vi "HFRR ADV v01.vi"() -> ()   [LabVIEW 2025] (continued)
                    n2104 = property on="Electrical Contact Resistance ( % )" class="WFChart (strict)"("History Data"=w3138) -> ()  [unwired: 2 in, 2 out]
                    n2105 = property on="Temperature ( Deg C )" class="WFChart (strict)"("History Data"=w3138) -> ()  [unwired: 2 in, 2 out]
                    n2106 = property on="Humidity ( %RH )" class="WFChart (strict)"("History Data"=w3138) -> ()  [unwired: 2 in, 2 out]
                    n2107 = property on="Stroke ( mm )" class="WFChart (strict)"("History Data"=w3139) -> ()  [unwired: 2 in, 2 out]
                    n2108 = property on="Stroke ( mm )" class="WFChart (strict)"("History Data"=w3139) -> ()  [unwired: 2 in, 2 out]
                    n2109 = local write "Humidity"(w3140) -> ()
                    n2110 = local write "Heater Button"(w3140) -> ()
                    n2111 = local read "FILE"() -> (w3134:string)
                    n2112 = disable-structure shown="Enabled" {
                      disable-tunnel: [w3179 _] -> w3125
                      frame Enabled {
                        n2113 = local read "NORMAL LOAD"() -> (w3179:dbl)
                      }
                      frame Disabled {
                      }
                    }
                    n2114 = call "file check.vi"("file name in"=w3134) -> ("error out"=w3137:errorcluster, "file name out"=w3131:string)  [unwired: 9 in]
                    n2115 = call "FILE PATH CREATION.vi"("error in"=w3137, "FILE NAME :"=w3131) -> ("FILE OUT"=w3130:path)  [unwired: 8 in, 1 out]
                    n2116 = Concatenate Strings(w3131, ".dgf" ("Substring")) -> (w3136:string)
                    n2117 = Concatenate Strings(w3131, ".duf" ("Substring")) -> (w3132:string)
                    n2118 = Multiply(x=w3125, y=1.0) -> (x*y=w3158:dbl)
                    n2119 = Build Path(base path=w3130, name or relative path=w3136) -> (appended path=w3129:path)
                    n2120 = Build Path(base path=w3130, name or relative path=w3132) -> (appended path=w3128:path)
                    n2121 = Number To Fractional String(number=w3158, width (-)=i16 5, precision (6)=i16 2) -> (F-format string=w3166:string)  [unwired: 1 in]
                    n2122 = local read "Fuel Discription :"() -> (w3154:string)
                    n2123 = local read "Batch Ref Num :"() -> (w3142:string)
                    n2124 = Get Date/Time String(date format (0)=enum16{"short", "long", "abbreviated"}."short") -> (date string=w3177:string, time string=w3174:string)  [unwired: 2 in]
                    n2125 = local read "Remarks :"() -> (w3153:string)
                    n2126 = Concatenate Strings("Load :- " ("Substring"), w3166, " grams ," ("Substring")) -> (w3165:string)
                    n2127 = local read "String 41"() -> (w3145:string)
                    n2128 = Concatenate Strings(w3154) -> (w3155:string)
                    n2129 = Concatenate Strings(w3142) -> (w3141:string)
                    n2130 = Concatenate Strings("tested by") -> (w3149:string)
                    n2131 = Concatenate Strings("(" ("Substring"), w3177, ")" ("Substring"), w3174) -> (w3147:string)
                    "concatenated string" <- w3147
                    n2132 = Concatenate Strings(w3153, "," ("string")) -> (w3152:string)
                    n2133 = Concatenate Strings("  TIME;      COF;       STROKE;     AIR TEMP;  TEMP;  HUMIDITY;  ECR; PID-OUT; FREQUENCY" ("Substring"), "\r") -> (w3161:string)
                    n2134 = Concatenate Strings(w3145, w3144, "Fuel Discription :-" ("Substring"), w3155, w3144, w3165, w3144, "Batch Ref Num :-" ("Substring"), w3141, w3144, " Remarks :- " ("Substring"), w3152, w3144, " Date :- " ("Substring"), w3147, w3144, "Tested By :-" ("Substring"), w3149) -> (w3159:string)
                    "REMARKS" <- w3159
                    n2135 = call <vilib>:"Write Characters To File.vi"("append to file? (new file:F)"=FALSE, "character string"=w3161, "file path (dialog if empty)"=w3129) -> ()  [unwired: 2 in, 1 out]
                    n2136 = call <vilib>:"Write Characters To File.vi"("append to file? (new file:F)"=FALSE, "character string"=w3159, "file path (dialog if empty)"=w3128) -> ()  [unwired: 2 in, 1 out]
                  }
                  frame #2 {
                    n2137 = local write "Cycles elapsed"(0 ("Cycles elapsed")) -> ()
                    n2138 = local write "cyclecount"(0 ("cyclecount")) -> ()
                    n2139 = local write "Save & Continue"(FALSE ("OK")) -> ()
                    n2140 = local write "autostrtflg"(TRUE ("autostrtflg")) -> ()
                    n2141 = local write "Save"(FALSE ("Save")) -> ()
                    n2142 = Get Date/Time In Seconds() -> (seconds since 1Jan1904=w3184:timestamp)
                    n2143 = To Double Precision Float(number=w3184) -> (double precision float=w3183:dbl)
                    n2144 = local write "acq timer"(w3183) -> ()
                    n2145 = One Button Dialog(message="Please ensure sample is mounted properly and machine is ready in all aspects for testing !", button name ("OK")="Ok") -> ()  [unwired: 1 out]
                  }
                  frame #3 {
                    n2146 = stacked-sequence {
                      frame #0 {
                        n2147 = local write "Main Dashboard Buttons"(T1."Dashboard" ("Main Dashboard Buttons")) -> ()
                        n2148 = local write "Main Tab"(T2."Acquire" ("Main Tab")) -> ()
                      }
                      frame #1 {
                        n2149 = local write "EVENT LOG"("" ("EVENT LOG")) -> ()
                      }
                      frame #2 {
                        n2150 = Wait (ms)(milliseconds to wait=u32 50) -> ()  [unwired: 1 out]
                      }
                      frame #3 {
                        n2151 = disable-structure shown="Disabled" {
                          frame Disabled {
                            n2152 = local read "EVENT LOG"() -> (w3196:string)
                            n2153 = call "Event Log.vi"("Content"="Test Details", "EVENT LOG"=w3196) -> ("EVENT LOG"=w3195:string)  [unwired: 8 in, 1 out]
                            n2154 = local write "EVENT LOG"(w3195) -> ()
                          }
                          frame Enabled {
                          }
                        }
                      }
                      frame #4 {
                        n2155 = Wait (ms)(milliseconds to wait=u32 50) -> ()  [unwired: 1 out]
                      }
                      frame #5 {
                        n2156 = local read "FILE"() -> (w3198:string)
                        n2157 = Concatenate Strings("File Name :" ("Content"), w3198) -> (w3199:string)
                        n2158 = local read "EVENT LOG"() -> (w3202:string)
                        n2159 = call "Event Log.vi"("Content"=w3199, "EVENT LOG"=w3202) -> ("EVENT LOG"=w3201:string)  [unwired: 8 in, 1 out]
                        n2160 = local write "EVENT LOG"(w3201) -> ()
                      }
                      frame #6 {
                        n2161 = Wait (ms)(milliseconds to wait=u32 50) -> ()  [unwired: 1 out]
                      }
                      frame #7 {
                        n2162 = local read "Batch Ref Num :"() -> (w3204:string)
                        n2163 = Concatenate Strings("Batch Ref No :" ("Content"), w3204) -> (w3205:string)
                        n2164 = local read "EVENT LOG"() -> (w3208:string)
                        n2165 = call "Event Log.vi"("Content"=w3205, "EVENT LOG"=w3208) -> ("EVENT LOG"=w3207:string)  [unwired: 8 in, 1 out]
                        n2166 = local write "EVENT LOG"(w3207) -> ()
                      }
                      frame #8 {
                        n2167 = Wait (ms)(milliseconds to wait=u32 50) -> ()  [unwired: 1 out]
                      }
                      frame #9 {
                        n2168 = local read "tested by"() -> (w3210:string)
                        n2169 = Concatenate Strings("Tested By :" ("Content"), w3210) -> (w3211:string)
                        n2170 = local read "EVENT LOG"() -> (w3214:string)
                        n2171 = call "Event Log.vi"("Content"=w3211, "EVENT LOG"=w3214) -> ("EVENT LOG"=w3213:string)  [unwired: 8 in, 1 out]
                        n2172 = local write "EVENT LOG"(w3213) -> ()
                      }
                      frame #10 {
                        n2173 = Wait (ms)(milliseconds to wait=u32 50) -> ()  [unwired: 1 out]
                      }
                      frame #11 {
                        n2174 = local read "TEST STANDARD"() -> (w3217:T3)
                        n2175 = case shown="\"ASTM D6079\", Default" w3217 {
                          tunnel: ["ASTM D6079" "ISO 12156" "CEC F-096-A-06" "Custom"] -> w3216
                          frame "ASTM D6079", Default {
                          }
                          frame "ISO 12156" {
                          }
                          frame "CEC F-096-A-06" {
                          }
                          frame "Custom" {
                          }
                        }
                        n2176 = Concatenate Strings("Test Standard :" ("Content"), w3216) -> (w3218:string)
                        n2177 = local read "EVENT LOG"() -> (w3221:string)
                        n2178 = call "Event Log.vi"("Content"=w3218, "EVENT LOG"=w3221) -> ("EVENT LOG"=w3220:string)  [unwired: 8 in, 1 out]
                        n2179 = local write "EVENT LOG"(w3220) -> ()
                      }
                      frame #12 {
                        n2180 = Wait (ms)(milliseconds to wait=u32 50) -> ()  [unwired: 1 out]
                      }
                      frame #13 {
                        n2181 = local read "Fuel Discription :"() -> (w3227:string)
                        n2182 = Concatenate Strings("Fuel Description :" ("Content"), w3227) -> (w3228:string)
                        n2183 = local read "EVENT LOG"() -> (w3231:string)
                        n2184 = call "Event Log.vi"("Content"=w3228, "EVENT LOG"=w3231) -> ("EVENT LOG"=w3230:string)  [unwired: 8 in, 1 out]
                        n2185 = local write "EVENT LOG"(w3230) -> ()
                      }
                      frame #14 {
                        n2186 = Wait (ms)(milliseconds to wait=u32 50) -> ()  [unwired: 1 out]
                      }
                      frame #15 {
                        n2187 = local read "Remarks :"() -> (w3233:string)
                        n2188 = Concatenate Strings("Remarks :" ("Content"), w3233) -> (w3234:string)
                        n2189 = local read "EVENT LOG"() -> (w3237:string)
                        n2190 = call "Event Log.vi"("Content"=w3234, "EVENT LOG"=w3237) -> ("EVENT LOG"=w3236:string)  [unwired: 8 in, 1 out]
                        n2191 = local write "EVENT LOG"(w3236) -> ()
                      }
                      frame #16 {
                        n2192 = Wait (ms)(milliseconds to wait=u32 50) -> ()  [unwired: 1 out]
                      }
                      frame #17 {
                        n2193 = local read "Operator ID"() -> (w3239:string)
                        n2194 = Concatenate Strings("Operator ID :" ("Content"), w3239) -> (w3241:string)
                        n2195 = local read "EVENT LOG"() -> (w3243:string)
                        n2196 = call "Event Log.vi"("Content"=w3241, "EVENT LOG"=w3243) -> ("EVENT LOG"=w3242:string)  [unwired: 8 in, 1 out]
                        n2197 = local write "EVENT LOG"(w3242) -> ()
                      }
                      frame #18 {
                        n2198 = Wait (ms)(milliseconds to wait=u32 50) -> ()  [unwired: 1 out]
                      }
                      frame #19 {
                        n2199 = disable-structure shown="Disabled" {
                          frame Disabled {
                            n2200 = local read "EVENT LOG"() -> (w3247:string)
                            n2201 = call "Event Log.vi"("Content"="Test Parameter", "EVENT LOG"=w3247) -> ("EVENT LOG"=w3246:string)  [unwired: 8 in, 1 out]
                            n2202 = local write "EVENT LOG"(w3246) -> ()
                          }
                          frame Enabled {
                          }
                        }
                      }
                      frame #20 {
                        n2203 = Wait (ms)(milliseconds to wait=u32 50) -> ()  [unwired: 1 out]
                      }
                      frame #21 {
                        n2204 = local read "Set Hz"() -> (w3251:dbl)
                        n2205 = Number To Fractional String(number=w3251, precision (6)=i16 2) -> (F-format string=w3250:string)  [unwired: 2 in]
                        n2206 = Concatenate Strings("Set Frequency [Hz] :" ("Content"), w3250) -> (w3253:string)
                        n2207 = local read "EVENT LOG"() -> (w3255:string)
                        n2208 = call "Event Log.vi"("Content"=w3253, "EVENT LOG"=w3255) -> ("EVENT LOG"=w3254:string)  [unwired: 8 in, 1 out]
                        n2209 = local write "EVENT LOG"(w3254) -> ()
                      }
                      frame #22 {
                        n2210 = Wait (ms)(milliseconds to wait=u32 50) -> ()  [unwired: 1 out]
                      }
                      frame #23 {
                        n2211 = local read "NORMAL LOAD"() -> (w3258:dbl)
                        n2212 = Number To Fractional String(number=w3258, precision (6)=i16 2) -> (F-format string=w3259:string)  [unwired: 2 in]
                        n2213 = Concatenate Strings("Applied Load [grams] :" ("Content"), w3259) -> (w3261:string)
                        n2214 = local read "EVENT LOG"() -> (w3263:string)
                        n2215 = call "Event Log.vi"("Content"=w3261, "EVENT LOG"=w3263) -> ("EVENT LOG"=w3262:string)  [unwired: 8 in, 1 out]
                        n2216 = local write "EVENT LOG"(w3262) -> ()
                      }
                      frame #24 {
                        n2217 = Wait (ms)(milliseconds to wait=u32 50) -> ()  [unwired: 1 out]
                      }
                      frame #25 {
                        n2218 = local read "Set Strk"() -> (w3266:dbl)
                        n2219 = Number To Fractional String(number=w3266, precision (6)=i16 2) -> (F-format string=w3267:string)  [unwired: 2 in]
                        n2220 = Concatenate Strings("Set Stroke [mm] :" ("Content"), w3267) -> (w3269:string)
                        n2221 = local read "EVENT LOG"() -> (w3271:string)
                        n2222 = call "Event Log.vi"("Content"=w3269, "EVENT LOG"=w3271) -> ("EVENT LOG"=w3270:string)  [unwired: 8 in, 1 out]
                        n2223 = local write "EVENT LOG"(w3270) -> ()
                      }
                      frame #26 {
                        n2224 = Wait (ms)(milliseconds to wait=u32 50) -> ()  [unwired: 1 out]
                      }
                      frame #27 {
                        n2225 = local read "Set Temp"() -> (w3274:dbl)
                        n2226 = Number To Fractional String(number=w3274, precision (6)=i16 2) -> (F-format string=w3275:string)  [unwired: 2 in]
                        n2227 = Concatenate Strings("Set Temperature [deg C] :" ("Content"), w3275) -> (w3277:string)
                        n2228 = local read "EVENT LOG"() -> (w3279:string)
                        n2229 = call "Event Log.vi"("Content"=w3277, "EVENT LOG"=w3279) -> ("EVENT LOG"=w3278:string)  [unwired: 8 in, 1 out]
                        n2230 = local write "EVENT LOG"(w3278) -> ()
                      }
                      frame #28 {
                        n2231 = Wait (ms)(milliseconds to wait=u32 50) -> ()  [unwired: 1 out]
                      }
                      frame #29 {
                        n2232 = local read "Set Rh"() -> (w3282:dbl)
                        n2233 = Number To Fractional String(number=w3282, precision (6)=i16 2) -> (F-format string=w3283:string)  [unwired: 2 in]
                        n2234 = Concatenate Strings("Set Humidity [%RH] :" ("Content"), w3283) -> (w3285:string)
                        n2235 = local read "EVENT LOG"() -> (w3287:string)
                        n2236 = call "Event Log.vi"("Content"=w3285, "EVENT LOG"=w3287) -> ("EVENT LOG"=w3286:string)  [unwired: 8 in, 1 out]
                        n2237 = local write "EVENT LOG"(w3286) -> ()
                      }
                      frame #30 {
                        n2238 = Wait (ms)(milliseconds to wait=u32 50) -> ()  [unwired: 1 out]
                      }
                      frame #31 {
                        n2239 = local read "test time"() -> (w3290:dbl)
                        n2240 = Number To Fractional String(number=w3290, precision (6)=i16 1) -> (F-format string=w3291:string)  [unwired: 2 in]
                        n2241 = Concatenate Strings("Test Duration [mins] :" ("Content"), w3291) -> (w3293:string)
                        n2242 = local read "EVENT LOG"() -> (w3295:string)
                        n2243 = call "Event Log.vi"("Content"=w3293, "EVENT LOG"=w3295) -> ("EVENT LOG"=w3294:string)  [unwired: 8 in, 1 out]
                        n2244 = local write "EVENT LOG"(w3294) -> ()
                      }
                      frame #32 {
                        w3296 = dbl[] [] ("History Data")
                        w3297 = cluster{"y":dbl, dbl, "y":dbl}[] [] ("History Data")
                        w3298 = FALSE ("Visible")
                        n2245 = property on="Stroke ( mm )" class="WFChart (strict)"("History Data"=w3297) -> ()  [unwired: 2 in, 2 out]
                        n2246 = property on="Humidity ( %RH )" class="WFChart (strict)"("History Data"=w3296) -> ()  [unwired: 2 in, 2 out]
                        n2247 = property on="Temperature ( Deg C )" class="WFChart (strict)"("History Data"=w3296) -> ()  [unwired: 2 in, 2 out]
                        n2248 = property on="Electrical Contact Resistance ( % )" class="WFChart (strict)"("History Data"=w3296) -> ()  [unwired: 2 in, 2 out]
                        n2249 = property on="Coefficient of Friction" class="WFChart (strict)"("History Data"=w3296) -> ()  [unwired: 2 in, 2 out]
                        n2250 = property on="Frictional Force ( N )" class="WFChart (strict)"("History Data"=w3296) -> ()  [unwired: 2 in, 2 out]
                        n2251 = property on="Coefficient of Friction" class="WFChart (strict)"("History Data"=w3296) -> ()  [unwired: 2 in, 2 out]
                        n2252 = property on="Frictional Force ( N )" class="WFChart (strict)"("History Data"=w3296) -> ()  [unwired: 2 in, 2 out]
                        n2253 = property on="Electrical Contact Resistance ( % )" class="WFChart (strict)"("History Data"=w3296) -> ()  [unwired: 2 in, 2 out]
                        n2254 = property on="Humidity ( %RH )" class="WFChart (strict)"("History Data"=w3296) -> ()  [unwired: 2 in, 2 out]
                        n2255 = property on="Stroke ( mm )" class="WFChart (strict)"("History Data"=w3297) -> ()  [unwired: 2 in, 2 out]
                        n2256 = property on="Temperature ( Deg C )" class="WFChart (strict)"("History Data"=w3296) -> ()  [unwired: 2 in, 2 out]
                        n2257 = property on="Service Password Log" class="Str"("Visible"=w3298) -> ()  [unwired: 2 in, 2 out]
                        n2258 = property on="Password 3" class="Clust (strict)"("Visible"=w3298) -> ()  [unwired: 2 in, 2 out]
                      }
                    }
                    "TEST FILE NAM,E SAVED" <- TRUE ("TEST FILE NAM,E SAVED")
                  }
                }
              }
            }
          }
        }
        n2259 = case shown="True" w2614 {
          frame False {
            n2260 = local write "tfalg"(0.0 ("tfalg")) -> ()
          }
          frame True {
            n2261 = local read "tfalg"() -> (w2759:dbl)
            n2262 = Equal?(x=w2759, y=0.0) -> (x = y?=w2760:bool)
            n2263 = case shown="True" w2760 {
              frame False {
              }
              frame True {
                n2264 = local read "Total No. of Tests"() -> (w2763:dbl)
                n2265 = local write "tfalg"(1.0 ("tfalg")) -> ()
                n2266 = local write "acq 2"(FALSE ("acq 2")) -> ()
                n2267 = Wait (ms)(milliseconds to wait=u32 200) -> ()  [unwired: 1 out]
                n2268 = Increment(x=w2763) -> (x+1=w2762:dbl)
                n2269 = local write "Total No. of Tests"(w2762) -> ()
              }
            }
          }
        }
        n2270 = local write "Test \nStatus"(w2620) -> ()
        n2271 = local write "Save"(w2620) -> ()
        n2272 = local read "Main Tab"() -> (w2577:T2)
        n2273 = case shown="True" w2601 {
          tunnel: [FALSE ("RUN") TRUE ("RUN")] -> w2600
          tunnel: [_ 1] -> w2593
          frame False {
          }
          frame True {
          }
        }
        n2274 = In Range and Coerce(upper limit=w2608, x=w2581, lower limit=w2607) -> (In Range?=w2599:bool)  [unwired: 1 out]
        n2275 = In Range and Coerce(upper limit=w2605, x=w2580, lower limit=w2606) -> (In Range?=w2597:bool)  [unwired: 1 out]
        n2276 = case shown="True" w2613 {
          frame False {
            n2277 = local read "Rt 3"() -> (w2741:bool)
            n2278 = case shown="True" w2741 {
              frame False {
              }
              frame True {
                n2279 = local write "Rt 3"(FALSE ("Rt 3")) -> ()
                n2280 = local write "Json End Flg"(TRUE ("Upld AR 2")) -> ()
              }
            }
            "Rt" <- TRUE ("Rt")
            "Rt 2" <- FALSE ("Rt")
          }
          frame True {
            n2281 = local read "Rt"() -> (w2748:bool)
            n2282 = local write "Rt 2"(TRUE ("Rt 2")) -> ()
            n2283 = case shown="True" w2748 {
              frame False {
              }
              frame True {
                w2749 = TRUE ("Upld AR 2")
                n2284 = local write "Rt"(FALSE ("Rt")) -> ()
                n2285 = local write "Upld AR"(w2749) -> ()
                n2286 = local write "Json St Flg"(w2749) -> ()
              }
            }
            "Rt 3" <- TRUE ("Rt 3")
          }
        }
        n2287 = case shown="True" w2599 {
          tunnel: [FALSE ("RUN") TRUE ("RUN")] -> w2598
          tunnel: [_ 2] -> w2592
          frame False {
          }
          frame True {
          }
        }
        n2288 = case shown="True" w2597 {
          tunnel: [FALSE ("RUN") TRUE ("RUN")] -> w2596
          tunnel: [_ 3] -> w2591
          frame False {
          }
          frame True {
          }
        }
        n2289 = case shown="\"Acquire\"" w2577 {
          tunnel: w2579 -> [_ w2810]
          frame Default {
            w2809 = 0.0 ("output")
            n2290 = local write "PID-out"(w2809) -> ()
            n2291 = local write "Frequency ( Hz )"(w2809) -> ()
          }
          frame "Acquire" {
            n2292 = stacked-sequence {
              frame #0 {
                n2293 = local read "Auto Start Test"() -> (w2812:bool)
                n2294 = case shown="True" w2812 {
                  tunnel: "RUN" -> [w2833 w2836]
                  tunnel: [w2833 w2835] -> w2813
                  frame False {
                  }
                  frame True {
                    n2295 = local read "Auto Start Temp"() -> (w2834:bool)
                    n2296 = Or(x=w2836, y=w2834) -> (x .or. y?=w2835:bool)
                  }
                }
                n2297 = local read "clk"() -> (w2832:dbl)
                n2298 = local read "Save"() -> (w2828:bool)
                n2299 = Equal?(x=w2832, y=0.0) -> (x = y?=w2829:bool)
                n2300 = And(x=w2829, y=w2828) -> (x .and. y?=w2830:bool)
                n2301 = Not(x="Engage") -> (.not. x?=w2819:bool)
                n2302 = case shown="False" w2813 {
                  tunnel: [0.0 w2860] -> w2815
                  frame False {
                    (unwired) TRUE ("Visible")
                    n2303 = local read "Auto Start Test"() -> (w2840:bool)
                    n2304 = local write "Start Time"(TRUE ("Start Time")) -> ()
                    n2305 = property on="Stroke 2" class="DigNum (strict)"("Visible"=FALSE) -> ()  [unwired: 2 in, 2 out]
                    n2306 = case shown="False" w2840 {
                      frame False {
                        n2307 = property on="Heater Button" class="Bool (strict)"("DisabledEnum"=T15."Enabled" ("Disabled")) -> ()  [unwired: 2 in, 2 out]
                        n2308 = property on="Humidity" class="Bool (strict)"("DisabledEnum"=T15."Enabled" ("Disabled")) -> ()  [unwired: 2 in, 2 out]
                      }
                      frame True {
                      }
                    }
                    n2309 = case shown="False" "TestCompFlg" {
                      frame False {
                        n2310 = local read "StartFlg"() -> (w2848:bool)
                        n2311 = case shown="True" w2848 {
                          frame False {
                          }
                          frame True {
                            n2312 = flat-sequence {
                              frame #0 {
                                n2313 = local read "EVENT LOG"() -> (w2850:string)
                                n2314 = call "Event Log.vi"("Content"="Test was interrupted", "EVENT LOG"=w2850) -> ("EVENT LOG"=w2851:string)  [unwired: 8 in, 1 out]
                                n2315 = local write "EVENT LOG"(w2851) -> ()
                              }
                              frame #1 {
                                w2852 = FALSE ("StartFlg")
                                n2316 = local write "Heater Button"(w2852) -> ()
                                n2317 = local write "StartFlg"(w2852) -> ()
                                n2318 = local write "Humidity"(w2852) -> ()
                              }
                            }
                          }
                        }
                      }
                      frame True {
                      }
                    }
                    n2319 = local write "String 14"("Test will autostart once parameters reach the set value." ("String 14")) -> ()
                  }
                  frame True {
                    (unwired) FALSE ("Visible")
                    n2320 = property on="Stroke 2" class="DigNum (strict)"("Visible"=TRUE) -> ()  [unwired: 2 in, 2 out]
                    n2321 = property on="STOP 2" class="Bool (strict)"("Disabled"=u8 2) -> ()  [unwired: 2 in, 2 out]
                    n2322 = local write "String 14"(" Running....." ("String 14")) -> ()
                    n2323 = property on="Heater Button" class="Bool (strict)"("DisabledEnum"=T15."Disabled and Grayed Out" ("Disabled")) -> ()  [unwired: 2 in, 2 out]
                    n2324 = property on="Humidity" class="Bool (strict)"("DisabledEnum"=T15."Disabled and Grayed Out" ("Disabled")) -> ()  [unwired: 2 in, 2 out]
                    n2325 = case shown="True" "Start Time" {
                      selector: "Start Time" -> [_ w2870]
                      frame False {
                      }
                      frame True {
                        n2326 = Not(x=w2870) -> (.not. x?=w2869:bool)
                        n2327 = local write "Start Time"(w2869) -> ()
                        n2328 = local read "EVENT LOG"() -> (w2871:string)
                        n2329 = call "Event Log.vi"("Content"="Test in progress", "EVENT LOG"=w2871) -> ("EVENT LOG"=w2873:string)  [unwired: 8 in, 1 out]
                        n2330 = local write "EVENT LOG"(w2873) -> ()
                      }
                    }
                    n2331 = local read "Set Hz"() -> (w2867:dbl)
                    n2332 = call <vilib>:"Uniform White Noise Waveform.vi"() -> ("signal out"=w2866:waveform(dbl))  [unwired: 10 in, 1 out]
                    n2333 = local read "Freq"() -> (w2859:dbl)
                    n2334 = Add(x=w2867, y=w2866) -> (x+y=w2865:waveform(dbl))
                    n2335 = Multiply(x=w2865, y=ext 0.1) -> (x*y=w2861:waveform(ext))
                    n2336 = Multiply(x=w2859, y=0.9) -> (x*y=w2862:dbl)
                    n2337 = Add(x=w2861, y=w2862) -> (x+y=w2860:waveform(ext))
                    "StartFlg" <- TRUE ("StartFlg")
                  }
                }
                n2338 = case shown="True" w2830 {
                  frame False {
                  }
                  frame True {
                    n2339 = local write "clk"(10.0 ("clk")) -> ()
                    n2340 = Get Date/Time In Seconds() -> (seconds since 1Jan1904=w2876:timestamp)
                    n2341 = To Double Precision Float(number=w2876) -> (double precision float=w2874:dbl)
                    n2342 = local write "acq timer"(w2874) -> ()
                    n2343 = local write "act save time"(w2874) -> ()
                  }
                }
                n2344 = call "Elapsed Time"("Time Target (s)"="Countdown", "Reset"=w2819) -> ("Elapsed Time (s)"=w2824:dbl, "Time has Elapsed"=w2822:bool)  [unwired: 10 in, 6 out]
                "Countdown 2" <- w2824
                n2345 = Subtract(x=w2824, y=2.0) -> (x-y=w2827:dbl)
                n2346 = Less?(x=w2827, y="Countdown") -> (x < y?=w2825:bool)
                n2347 = And(x=w2825, y=w2822) -> (x .and. y?=w2821:bool)
                n2348 = case shown="True" w2821 {
                  frame False {
                  }
                  frame True {
                    (unwired) dbl[] [] ("History Data")
                    n2349 = local write "Engage"(FALSE ("Engage")) -> ()
                    n2350 = local write "RUN"(TRUE ("RUN")) -> ()
                    n2351 = local read "Humidity ( %RH )"() -> (→"Rh Before":dbl)
                  }
                }
                n2352 = local read "Test \nStatus"() -> (w2817:bool)
                n2353 = Select(t=w2815, s=w2817, f=0.0) -> (s? t:f=w2816:dbl)
                n2354 = local write "Frequency ( Hz )"(w2816) -> ()
                n2355 = local write "Freq"(w2816) -> ()
              }
              frame #1 {
                w2899 = 1000000.0 ("x")
                # "Elapsed time\ncof\nstroke\nAir temp\nTemp\nHumidity"
                # "acq timer\n\nact save time"
                # "convert to microseconds"
                n2356 = local read "COUNT"() -> (w2882:i32)
                n2357 = local read "Rate"() -> (w2895:dbl)
                n2358 = Divide(x=w2899, y=w2895) -> (x/y=w2900:dbl)
                n2359 = Greater Or Equal?(x=w2882, y=250) -> (x >= y?=w2881:bool)
                n2360 = Get Date/Time In Seconds() -> (seconds since 1Jan1904=w2902:timestamp)
                n2361 = case shown="True" w2881 {
                  frame False {
                    n2362 = local read "COUNT"() -> (w2903:i32)
                    n2363 = Increment(x=w2903) -> (x+1=w2904:i32)
                    n2364 = local write "COUNT"(w2904) -> ()
                  }
                  frame True {
                    n2365 = local write "COUNT"(0 ("COUNT")) -> ()
                  }
                }
                n2366 = local read "Samplingtime 2"() -> (w2880:dbl)
                n2367 = local read "act save time"() -> (w2897:dbl)
                n2368 = Divide(x=w2900, y=w2899) -> (x/y=w2898:dbl)
                n2369 = To Double Precision Float(number=w2902) -> (double precision float=w2891:dbl)
                n2370 = Add(x=w2897, y=w2880) -> (x+y=w2896:dbl)
                n2371 = local read "acq timer"() -> (w2901:dbl)
                n2372 = local read "COUNT"() -> (w2884:i32)
                n2373 = Greater Or Equal?(x=w2891, y=w2896) -> (x >= y?=w2879:bool)
                n2374 = Multiply(x=w2898, y=w2884) -> (x*y=w2890:dbl)
                n2375 = Subtract(x=w2891, y=w2901) -> (x-y=w2893:dbl)
                n2376 = local read "Save"() -> (w2894:bool)
                n2377 = Add(x=w2893, y=w2890) -> (x+y=w2877:dbl)
                "Elapsed time 3" <- w2877
                n2378 = And(x=w2879, y=w2894) -> (x .and. y?=w2892:bool)
                n2379 = Divide(x=w2877, y=60.0) -> (x/y=w2888:dbl)
                n2380 = local read "Test \nStatus"() -> (w2878:bool)
                n2381 = local read "clk"() -> (w2885:dbl)
                n2382 = Equal?(x=w2885, y=10.0) -> (x = y?=w2887:bool)
                n2383 = case shown="True" w2892 {
                  tunnel: w2891 -> [_ w3001]
                  tunnel: [FALSE ("Boolean 2") TRUE ("Boolean 2")] -> _
                  frame False {
                  }
                  frame True {
                    w2955 = ";" ("Substring")
                    # "Pid out/\nFreq response value"
                    n2384 = local write "act save time"(w3001) -> ()
                    n2385 = local read "FILE"() -> (w2949:string)
                    n2386 = call "file check.vi"("file name in"=w2949) -> ("error out"=w2952:errorcluster, "file name out"=w2947:string)  [unwired: 9 in]
                    n2387 = call "FILE PATH CREATION.vi"("error in"=w2952, "FILE NAME :"=w2947) -> ("FILE OUT"=w2950:path)  [unwired: 8 in, 1 out]
                    n2388 = Concatenate Strings(w2947, ".dgf" ("Substring")) -> (w2951:string)
                    n2389 = local read "FF 2"() -> (→"Frictional Force ( N )" →"Frictional Force ( N )":dbl)
                    n2390 = Build Path(base path=w2950, name or relative path=w2951) -> (appended path=w2946:path)
                    n2391 = local read "COF 2"() -> (w2960:dbl)
                    "cof" <- w2960
                    "Coefficient of Friction" <- w2960
                    "COF 4" <- w2960
                    "Coefficient of Friction" <- w2960
                    n2392 = local read "TEMP"() -> (w2963:dbl)
                    "Temp" <- w2963
                    "Temperature ( Deg C )" <- w2963
                    n2393 = local read "Humidity ( %RH )"() -> (w2962:dbl)
                    "Humidity ( %RH )" <- w2962
                    "Humidity ( %RH )" <- w2962
                    n2394 = local read "Frequency ( Hz )"() -> (w2969:dbl)
                    n2395 = local read "Elapsed time"() -> (w2994:dbl)
                    n2396 = local read "AIR TEMP"() -> (w2967:dbl)
                    n2397 = local read "PID-out"() -> (w2972:dbl)
                    n2398 = local write "Temperature ( Deg C )"(w2963) -> ()
                    n2399 = Number To Fractional String(number="measured_stroke", width (-)=i16 9 ("precision (6)"), precision (6)=i16 6) -> (F-format string=w2987:string)  [unwired: 1 in]
                    n2400 = Number To Fractional String(number=w2967, width (-)=i16 9 ("precision (6)"), precision (6)=i16 3) -> (F-format string=w2986:string)  [unwired: 1 in]
                    n2401 = Number To Fractional String(number=w2963, width (-)=i16 9 ("precision (6)"), precision (6)=i16 3) -> (F-format string=w2983:string)  [unwired: 1 in]
                    n2402 = Number To Fractional String(number=w2962, width (-)=i16 9 ("precision (6)"), precision (6)=i16 3) -> (F-format string=w2980:string)  [unwired: 1 in]
                    n2403 = Number To Fractional String(number=0.0, width (-)=i16 9 ("precision (6)"), precision (6)=i16 3) -> (F-format string=w2977:string)  [unwired: 1 in]
                    n2404 = Number To Fractional String(number=w2972, width (-)=i16 9 ("precision (6)"), precision (6)=i16 3) -> (F-format string=w2973:string)  [unwired: 1 in]
                    n2405 = Number To Fractional String(number=w2969, width (-)=i16 9 ("precision (6)"), precision (6)=i16 3) -> (F-format string=w2968:string)  [unwired: 1 in]
                    n2406 = Number To Fractional String(number=w2960, width (-)=i16 9 ("precision (6)"), precision (6)=i16 6) -> (F-format string=w2995:string)  [unwired: 1 in]
                    n2407 = Number To Fractional String(number=w2994, width (-)=i16 14 ("precision (6)"), precision (6)=i16 3) -> (F-format string=w2996:string)  [unwired: 1 in]
                    n2408 = Bundle("y"=1.02, "measured_stroke"="measured_stroke", "y"=0.98) -> (w2961:cluster{"y":dbl, "measured_stroke":dbl, "y":dbl})  [unwired: 1 in]
                    n2409 = Number To Fractional String(number="Ambient Humidity :", width (-)=i16 9 ("precision (6)"), precision (6)=i16 6) -> (F-format string=w2953:string)  [unwired: 1 in]
                    n2410 = local read "RUN"() -> (w2959:bool)
                    n2411 = case shown="True" w2959 {
                      tunnel: w2961 -> [_ w3006]
                      tunnel: "measured_stroke" -> [_ w3005]
                      tunnel: "measured_stroke" -> [_ w3004]
                      tunnel: "measured_stroke" -> [_ w3003]
                      frame False {
                      }
                      frame True {
                        "Stroke ( mm )" <- w3006
                        "Stroke ( mm )" <- w3006
                        "Stroke 4" <- w3005
                        "Stroke 3" <- w3004
                        "Stroke 2" <- w3003
                      }
                    }
                    n2412 = Concatenate Strings(w2996, w2955, w2995, w2955, w2987, w2955, w2986, w2955, w2983, w2955, w2980, w2955, w2977, w2955, w2973, w2955, w2968, w2955, w2953, "\r") -> (w2993:string)
                    n2413 = call <vilib>:"Write Characters To File.vi"("append to file? (new file:F)"=TRUE, "character string"=w2993, "file path (dialog if empty)"=w2946) -> ()  [unwired: 2 in, 1 out]
                    "refresh flag" <- TRUE ("refresh flag")
                  }
                }
                n2414 = case shown="True" w2878 {
                  tunnel: w2888 -> [_ w2914]
                  tunnel: w2893 -> [_ w2924]
                  tunnel: [0.0 w2920] -> _
                  tunnel: w2887 -> [_ w2919]
                  tunnel: [0.0 w2918] -> _
                  tunnel: w2877 -> [_ w2918]
                  tunnel: w2891 -> [w2907 _]
                  frame False {
                    n2415 = local write "acq timer"(w2907) -> ()
                    n2416 = local write "Test Duration Status"(0.0 ("Test Duration Status")) -> ()
                  }
                  frame True {
                    n2417 = local read "Set Hz"() -> (w2921:dbl)
                    n2418 = local write "Elapsed time"(w2914) -> ()
                    n2419 = local read "test time"() -> (w2913:dbl)
                    n2420 = Multiply(x=w2924, y=w2921) -> (x*y=w2923:dbl)
                    n2421 = case shown="False" w2919 {
                      tunnel: w2923 -> [w2925 _]
                      tunnel: [w2925 1.0] -> w2920
                      frame False {
                        n2422 = local write "Cycles elapsed"(w2925) -> ()
                      }
                      frame True {
                      }
                    }
                    n2423 = Greater?(x=w2914, y=w2913) -> (0:w2922:bool)
                    n2424 = Subtract(x=w2913, y=w2914) -> (x-y=w2912:dbl)
                    "time" <- w2912
                    n2425 = Multiply(x=w2912, y=60.0) -> (x*y=w2911:dbl)
                    n2426 = local write "Time Remaining"(w2911) -> ()
                    n2427 = local write "Remaining Time"(w2911) -> ()
                    n2428 = case shown="True" w2922 {
                      frame False {
                      }
                      frame True {
                        w2927 = T15."Enabled" ("Disabled")
                        w2931 = "" ("FILE")
                        w2932 = TRUE ("Visible")
                        n2429 = local write "Humidity"(FALSE ("Humidity")) -> ()
                        n2430 = local write "RUN"(FALSE ("OK Button 2")) -> ()
                        n2431 = local write "Heater Button"(FALSE ("Heater Button")) -> ()
                        n2432 = local write "Auto Start Test"(FALSE ("Auto Start Test")) -> ()
                        n2433 = local write "TestCompFlg"(TRUE ("StpFlg")) -> ()
                        n2434 = local read "Humidity ( %RH )"() -> (→"Rh After":dbl)
                        n2435 = property on="STOP 2" class="Bool (strict)"("Disabled"=u8 0) -> ()  [unwired: 2 in, 2 out]
                        n2436 = local read "EVENT LOG"() -> (w2937:string)
                        n2437 = call "Event Log.vi"("Content"="Test Completed", "EVENT LOG"=w2937) -> ("EVENT LOG"=w2936:string)  [unwired: 8 in, 1 out]
                        n2438 = property on="RUN" class="Bool (strict)"("Visible"=w2932) -> ()  [unwired: 2 in, 2 out]
                        n2439 = property on="Auto Start Test" class="Bool (strict)"("Visible"=w2932) -> ()  [unwired: 2 in, 2 out]
                        n2440 = local write "Batch Ref Num :"(w2931) -> ()
                        n2441 = local write "FILE"(w2931) -> ()
                        n2442 = local write "EVENT LOG"(w2936) -> ()
                        n2443 = local write "TEST FILE NAM,E SAVED"(FALSE ("TEST FILE NAM,E SAVED")) -> ()
                        n2444 = local write "Fuel Discription :"(w2931) -> ()
                        n2445 = local write "Remarks :"(w2931) -> ()
                        n2446 = local write "Main Dashboard Buttons"(T1."Imaging" ("Main Dashboard Buttons")) -> ()
                        n2447 = local write "Main Tab"(T2."Adv Scar" ("Main Tab")) -> ()
                        n2448 = property on="FRICVALZ 2" class="Bool (strict)"("DisabledEnum"=w2927) -> ()  [unwired: 2 in, 2 out]
                        n2449 = property on="FRICVALZ 3" class="Bool (strict)"("DisabledEnum"=w2927) -> ()  [unwired: 2 in, 2 out]
                        n2450 = property on="FRICVALZ 4" class="Bool (strict)"("DisabledEnum"=w2927) -> ()  [unwired: 2 in, 2 out]
                      }
                    }
                    n2451 = Divide(x=w2914, y=w2913) -> (x/y=w2917:dbl)
                    n2452 = Multiply(x=w2917, y=100.0) -> (x*y=w2915:dbl)
                    n2453 = local write "Test Duration Status"(w2915) -> ()
                  }
                }
              }
              frame #2 {
                n2454 = case shown="True" "Heater Button" {
                  tunnel: [0.0 ("output") w3030] -> w3007
                  frame False {
                    w3010 = TRUE ("tmpchk")
                    n2455 = local read "TEMP"() -> (w3011:dbl)
                    n2456 = local write "Temp ini"(w3011) -> ()
                    n2457 = local write "Reset 4"(w3010) -> ()
                    n2458 = local write "tmpchk"(w3010) -> ()
                    n2459 = local write "reinit"(TRUE ("reinit")) -> ()
                    n2460 = local write "manual temp log"(TRUE ("manual temp log")) -> ()
                  }
                  frame True {
                    # "Logic to turn off\nthe heater when \ntemp is not rising.\nTime - 60 sec\nDelta t- 5°c"
                    n2461 = local read "Temp ini"() -> (w3018:dbl)
                    n2462 = local read "Auto Start Test"() -> (w3014:bool)
                    n2463 = Less?(x=w3018, y=53.0) -> (x < y?=w3016:bool)
                    n2464 = case shown="False" w3014 {
                      frame False {
                        n2465 = local read "Set Temp"() -> (w3041:dbl)
                        n2466 = local read "TEMP"() -> (w3040:dbl)
                        n2467 = Subtract(x=w3041, y=w3040) -> (x-y=w3039:dbl)
                        n2468 = Absolute Value(x=w3039) -> (abs(x)=w3038:dbl)
                        n2469 = Less?(x=w3038, y=0.5) -> (x < y?=w3036:bool)
                        n2470 = case shown="True" w3036 {
                          tunnel: "manual temp log" -> [_ w3042]
                          frame False {
                          }
                          frame True {
                            n2471 = case shown="True" w3042 {
                              selector: w3042 -> [_ w3043]
                              frame False {
                              }
                              frame True {
                                # "#Event log"
                                n2472 = Not(x=w3043) -> (.not. x?=w3044:bool)
                                n2473 = local write "manual temp log"(w3044) -> ()
                                n2474 = local read "EVENT LOG"() -> (w3047:string)
                                n2475 = call "Event Log.vi"("Content"="Target Temperature reached", "EVENT LOG"=w3047) -> ("EVENT LOG"=w3046:string)  [unwired: 8 in, 1 out]
                                n2476 = local write "EVENT LOG"(w3046) -> ()
                              }
                            }
                          }
                        }
                      }
                      frame True {
                        n2477 = local write "manual temp log"(TRUE ("manual temp log")) -> ()
                      }
                    }
                    n2478 = And(x="tmpchk", y=w3016) -> (x .and. y?=w3019:bool)
                    n2479 = case shown="True" w3019 {
                      frame False {
                      }
                      frame True {
                        n2480 = call "Elapsed Time8"("Time Target (s)"=300.0, "Reset"="Reset 4") -> ("Time has Elapsed"=w3049:bool)  [unwired: 10 in, 7 out]
                        n2481 = flat-sequence {
                          tunnel: w3049 -> [_]
                          frame #0 {
                            n2482 = local write "Reset 4"(FALSE ("Reset 4")) -> ()
                          }
                        }
                        n2483 = case shown="True" w3049 {
                          frame False {
                          }
                          frame True {
                            n2484 = local read "Temp ini"() -> (w3056:dbl)
                            n2485 = Add(x=w3056, y=5.0) -> (x+y=w3054:dbl)
                            n2486 = local read "TEMP"() -> (w3057:dbl)
                            n2487 = Greater?(x=w3057, y=w3054) -> (0:w3055:bool)
                            n2488 = case shown="False" w3055 {
                              frame False {
                                n2489 = local write "Heater Button"(FALSE ("Heater Button")) -> ()
                              }
                              frame True {
                                n2490 = local write "tmpchk"(FALSE ("tmpchk")) -> ()
                              }
                            }
                          }
                        }
                      }
                    }
                    n2491 = local read "Set Temp"() -> (w3027:dbl)
                    n2492 = local read "TEMP"() -> (w3021:dbl)
                    n2493 = call-poly <vilib>:"PID.vi"("reinitialize? (F)"="reinit", "output range"="output range", "dt (s)"=-1.0, "PID gains"="Temp PID gains", "process variable"=w3021, "setpoint"=w3027) -> ("output"=w3024:dbl)  [unwired: 4 in, 1 out]
                    n2494 = Subtract(x=w3027, y=w3021) -> (x-y=w3029:dbl)
                    n2495 = Add(x=w3027, y=0.5) -> (x+y=w3025:dbl)
                    n2496 = Greater Or Equal?(x=w3021, y=w3025) -> ()  [unwired: 1 out]
                    n2497 = Select(t=0.0, s=FALSE, f=w3024) -> (s? t:f=w3023:dbl)
                    "PID output" <- w3023
                    n2498 = flat-sequence {
                      tunnel: w3023 -> [w3060]
                      tunnel: [w3060] -> w3030
                      frame #0 {
                        n2499 = local write "reinit"(FALSE ("reinit")) -> ()
                      }
                    }
                    n2500 = Bundle(w3029, "output"=w3023, "TEMP"=w3021) -> (→"gTEMP 3":cluster{dbl, "output":dbl, "TEMP":dbl})  [unwired: 1 in]
                  }
                }
                "PID-out" <- w3007
              }
              frame #3 {
                n2501 = local read "TEMP"() -> (w3062:dbl)
                n2502 = Greater Or Equal?(x=w3062, y="Set Temp 2") -> (x >= y?=w3067:bool)
                n2503 = case shown="True" w3067 {
                  tunnel: [FALSE TRUE] -> w3065
                  frame False {
                  }
                  frame True {
                  }
                }
                "Status 13" <- w3065
                n2504 = And(x=w3065, y="trip1 8") -> (x .and. y?=w3064:bool)
                n2505 = case shown="True" w3064 {
                  frame False {
                    n2506 = local write "Heater Trip Temp"(TRUE ("Heater Trip Temp")) -> ()
                  }
                  frame True {
                    w3070 = FALSE ("OK Button 2")
                    n2507 = case shown="True" "Heater Trip Temp" {
                      selector: "Heater Trip Temp" -> [_ w3072]
                      frame False {
                      }
                      frame True {
                        n2508 = Not(x=w3072) -> (.not. x?=w3071:bool)
                        n2509 = local read "EVENT LOG"() -> (w3075:string)
                        n2510 = local write "Heater Trip Temp"(w3071) -> ()
                        n2511 = call "Event Log.vi"("Content"="Heater Trip", "EVENT LOG"=w3075) -> ("EVENT LOG"=w3074:string)  [unwired: 8 in, 1 out]
                        n2512 = local write "EVENT LOG"(w3074) -> ()
                      }
                    }
                    n2513 = local write "RUN"(w3070) -> ()
                    n2514 = property on="Auto Start Test" class="Bool (strict)"("Value"=w3070) -> ()  [unwired: 2 in, 2 out]
                    n2515 = local write "Heater Button"(w3070) -> ()
                  }
                }
              }
            }
            n2516 = case shown="False" w2810 {
              frame False {
                n2517 = disable-structure shown="Enabled" {
                  frame Enabled {
                    n2518 = stacked-sequence {
                      frame #0 {
                        n2519 = local write "RUN"(FALSE ("OK Button 2")) -> ()
                      }
                      frame #1 {
                      }
                    }
                  }
                  frame Disabled {
                  }
                }
              }
              frame True {
              }
            }
          }
        }
        n2520 = local read "airtempflg"() -> (w2602:bool)
        n2521 = Or(x=w2602, y=w2600) -> (x .or. y?=w2603:bool)
        n2522 = Insert Into Array(array=string[] ["Air Temperature has reached set value,", "Humidity has reached set value,", "Sample Temperaturehas reached set value,", ""], index=0, new element="") -> (w2588:string[])
        n2523 = Build Array(w2593, w2592, w2591) -> (w2589:i32[])
        n2524 = disable-structure shown="Disabled" {
          disable-tunnel: w2603 -> [w2680 _]
          disable-tunnel: w2598 -> [w2679 _]
          disable-tunnel: w2596 -> [w2678 _]
          frame Disabled {
            n2525 = Compound Arithmetic op=AND(w2680, w2679, w2678) -> ()  [unwired: 1 out]
            n2526 = case shown="True" {
              selector: _ -> [_ _]
              frame False {
              }
              frame True {
                w2681 = FALSE ("autostrtflg")
                n2527 = local write "RUN"(TRUE ("RUN")) -> ()
                n2528 = local write "autostrtflg"(w2681) -> ()
                n2529 = local write "autostart"(w2681) -> ()
                n2530 = local write "String 14"(" Running....." ("String 14")) -> ()
              }
            }
          }
          frame Enabled {
          }
        }
        n2531 = for {
          tunnel: w2589 -> [w2731] mode=indexing
          tunnel: w2588 -> [w2730]
          shift-right: [w2727] -> w2587
          shift-left: "" -> [w2729]
          n2532 = Index Array(array=w2730, index=w2731) -> (element=w2728:string)
          n2533 = Concatenate Strings(w2728, w2729) -> (w2727:string)
        }
        n2534 = local write "autostart 2"(w2587) -> ()
        n2535 = local read "Reset Graph"() -> (w2576:bool)
        n2536 = case shown="True" w2576 {
          selector: w2576 -> [_ w2630]
          frame False {
          }
          frame True {
            w2644 = 0.0 ("X Scale.Range:Maximum")
            n2537 = Not(x=w2630) -> (.not. x?=w2629:bool)
            n2538 = local write "Reset Graph"(w2629) -> ()
            n2539 = property on="Electrical Contact Resistance ( % )" class="WFChart (strict)"("XScale.Maximum"=600.0 ("X Scale.Range:Maximum"), "XScale.Minimum"=0.0 ("X Scale.Range:Minimum"), "YScale.Maximum"=100.0 ("Y Scale.Range:Maximum"), "YScale.Minimum"=0.0 ("Y Scale.Range:Minimum")) -> ()  [unwired: 2 in, 2 out]
            n2540 = property on="Frictional Force ( N )" class="WFChart (strict)"("XScale.Maximum"=600.0 ("X Scale.Range:Maximum"), "XScale.Minimum"=0.0 ("X Scale.Range:Minimum"), "YScale.Maximum"=100.0 ("Y Scale.Range:Maximum"), "YScale.Minimum"=0.0 ("Y Scale.Range:Minimum")) -> ()  [unwired: 2 in, 2 out]
            n2541 = property on="Temperature ( Deg C )" class="WFChart (strict)"("XScale.Maximum"=600.0 ("X Scale.Range:Maximum"), "XScale.Minimum"=0.0 ("X Scale.Range:Minimum"), "YScale.Maximum"=100.0 ("Y Scale.Range:Maximum"), "YScale.Minimum"=0.0 ("Y Scale.Range:Minimum")) -> ()  [unwired: 2 in, 2 out]
            n2542 = property on="Humidity ( %RH )" class="WFChart (strict)"("XScale.Maximum"=600.0 ("X Scale.Range:Maximum"), "XScale.Minimum"=0.0 ("X Scale.Range:Minimum"), "YScale.Maximum"=100.0 ("Y Scale.Range:Maximum"), "YScale.Minimum"=0.0 ("Y Scale.Range:Minimum")) -> ()  [unwired: 2 in, 2 out]
            n2543 = property on="Stroke ( mm )" class="WFChart (strict)"("XScale.Maximum"=600.0 ("X Scale.Range:Maximum"), "XScale.Minimum"=0.0 ("X Scale.Range:Minimum"), "YScale.Maximum"=100.0 ("Y Scale.Range:Maximum"), "YScale.Minimum"=0.0 ("Y Scale.Range:Minimum")) -> ()  [unwired: 2 in, 2 out]
            n2544 = property on="Coefficient of Friction" class="WFChart (strict)"("XScale.Maximum"=600.0 ("X Scale.Range:Maximum"), "XScale.Minimum"=0.0 ("X Scale.Range:Minimum"), "YScale.Maximum"=100.0 ("Y Scale.Range:Maximum"), "YScale.Minimum"=0.0 ("Y Scale.Range:Minimum")) -> ()  [unwired: 2 in, 2 out]
            n2545 = property on="Electrical Contact Resistance ( % )" class="WFChart (strict)"("XScale.Minimum"=0.0 ("X Scale.Range:Minimum"), "XScale.Maximum"=600.0 ("X Scale.Range:Maximum"), "YScale.Minimum"=0.0 ("Y Scale.Range:Minimum"), "YScale.Maximum"=100.0 ("Y Scale.Range:Maximum")) -> ()  [unwired: 2 in, 2 out]
            n2546 = property on="Temperature ( Deg C )" class="WFChart (strict)"("XScale.Minimum"=0.0 ("X Scale.Range:Minimum"), "XScale.Maximum"=600.0 ("X Scale.Range:Maximum"), "YScale.Minimum"=0.0 ("Y Scale.Range:Minimum"), "YScale.Maximum"=100.0 ("Y Scale.Range:Maximum")) -> ()  [unwired: 2 in, 2 out]
            n2547 = property on="Coefficient of Friction" class="WFChart (strict)"("XScale.Minimum"=0.0 ("X Scale.Range:Minimum"), "XScale.Maximum"=600.0 ("X Scale.Range:Maximum"), "YScale.Maximum"=1.0 ("X Scale.Range:Minimum"), "YScale.Minimum"=0.0 ("X Scale.Range:Minimum")) -> ()  [unwired: 2 in, 2 out]
            n2548 = property on="Frictional Force ( N )" class="WFChart (strict)"("XScale.Maximum"=600.0 ("X Scale.Range:Maximum"), "XScale.Minimum"=w2644, "YScale.Maximum"=10.0 ("Y Scale.Range:Maximum"), "YScale.Minimum"=w2644) -> ()  [unwired: 2 in, 2 out]
            n2549 = property on="Stroke ( mm )" class="WFChart (strict)"("XScale.Maximum"=600.0 ("X Scale.Range:Maximum"), "XScale.Minimum"=0.0 ("X Scale.Range:Minimum"), "YScale.Maximum"=100.0 ("Y Scale.Range:Maximum"), "YScale.Minimum"=0.0 ("Y Scale.Range:Minimum")) -> ()  [unwired: 2 in, 2 out]
            n2550 = property on="Humidity ( %RH )" class="WFChart (strict)"("XScale.Maximum"=600.0 ("X Scale.Range:Maximum"), "XScale.Minimum"=0.0 ("X Scale.Range:Minimum"), "YScale.Maximum"=100.0 ("Y Scale.Range:Maximum"), "YScale.Minimum"=0.0 ("Y Scale.Range:Minimum")) -> ()  [unwired: 2 in, 2 out]
          }
        }
      }
      frame "Compare Files" {
        # "Elapsed time\ncof\nstroke\nAir temp\nTemp\nHumidity"
        n2551 = case shown="True" "RSTV1 2" {
          frame False {
          }
          frame True {
            n2552 = property on="Humidity ( %RH )" class="XYGraph (strict)"("Y Scale.Display Format:Precision"=u8 0 ("Y Scale.Format & Precision:Precision")) -> ()  [unwired: 2 in, 2 out]
            n2553 = property on="Humidity ( %RH )" class="XYGraph (strict)"("X Scale.Range:Minimum"=0.0, "X Scale.Range:Maximum"=75.0, "Y Scale.Range:Minimum"=48.0, "Y Scale.Range:Maximum"=58.0) -> ()  [unwired: 2 in, 2 out]
          }
        }
        n2554 = case shown="True" "RST CP 2" {
          frame False {
          }
          frame True {
            n2555 = property on="XY Graph 13" class="XYGraph (strict)"("Y Scale.Display Format:Precision"=u8 0 ("Y Scale.Format & Precision:Precision")) -> ()  [unwired: 2 in, 2 out]
            n2556 = property on="XY Graph 13" class="XYGraph (strict)"("X Scale.Range:Minimum"=0.0, "X Scale.Range:Maximum"=75.0, "Y Scale.Range:Minimum"=0.0, "Y Scale.Range:Maximum"=100.0) -> ()  [unwired: 2 in, 2 out]
          }
        }
        n2557 = case shown="True" "RST CP" {
          frame False {
          }
          frame True {
            n2558 = property on="Sample Temperature ( °C )" class="XYGraph (strict)"("Y Scale.Display Format:Precision"=u8 2 ("Y Scale.Format & Precision:Precision")) -> ()  [unwired: 2 in, 2 out]
            n2559 = property on="Sample Temperature ( °C )" class="XYGraph (strict)"("X Scale.Range:Minimum"=0.0, "X Scale.Range:Maximum"=75.0, "Y Scale.Range:Minimum"=58.0, "Y Scale.Range:Maximum"=62.0) -> ()  [unwired: 2 in, 2 out]
          }
        }
        n2560 = case shown="True" "RSTV1 3" {
          frame False {
          }
          frame True {
            n2561 = property on="Air Temperature  ( °C )" class="XYGraph (strict)"("Y Scale.Display Format:Precision"=u8 2 ("Y Scale.Format & Precision:Precision")) -> ()  [unwired: 2 in, 2 out]
            n2562 = property on="Air Temperature  ( °C )" class="XYGraph (strict)"("X Scale.Range:Minimum"=0.0 ("Y Scale.Range:Minimum"), "X Scale.Range:Maximum"=75.0 ("Y Scale.Range:Maximum"), "Y Scale.Range:Minimum"=20.0 ("X Scale.Range:Minimum"), "Y Scale.Range:Maximum"=26.0 ("X Scale.Range:Maximum")) -> ()  [unwired: 2 in, 2 out]
          }
        }
        n2563 = case shown="True" "RSTV1 4" {
          frame False {
          }
          frame True {
            n2564 = property on="Stroke ( mm )" class="XYGraph (strict)"("Y Scale.Display Format:Precision"=u8 2 ("Y Scale.Format & Precision:Precision")) -> ()  [unwired: 2 in, 2 out]
            n2565 = property on="Stroke ( mm )" class="XYGraph (strict)"("X Scale.Range:Minimum"=0.0 ("Y Scale.Range:Maximum"), "X Scale.Range:Maximum"=75.0 ("X Scale.Range:Minimum"), "Y Scale.Range:Minimum"=0.98, "Y Scale.Range:Maximum"=1.02) -> ()  [unwired: 2 in, 2 out]
          }
        }
        n2566 = case shown="True" "rstv2" {
          frame False {
          }
          frame True {
            n2567 = property on="Coefficient Of Friction" class="XYGraph (strict)"("Y Scale.Display Format:Precision"=u8 3 ("Y Scale.Format & Precision:Precision")) -> ()  [unwired: 2 in, 2 out]
            n2568 = property on="Coefficient Of Friction" class="XYGraph (strict)"("X Scale.Range:Minimum"=0.0 ("Y Scale.Range:Maximum"), "X Scale.Range:Maximum"=75.0, "Y Scale.Range:Minimum"=0.0, "Y Scale.Range:Maximum"=1.0 ("X Scale.Range:Minimum")) -> ()  [unwired: 2 in, 2 out]
          }
        }
        n2569 = case shown="True" "RST CP 3" {
          frame False {
          }
          frame True {
            n2570 = property on="Air Temp ( °C ) vs Humidity ( % RH )" class="XYGraph (strict)"("X Scale.Range:Minimum"=18.0, "X Scale.Range:Maximum"=28.0 ("X Scale.Range:Minimum"), "Y Scale.Range:Minimum"=30.0 ("X Scale.Range:Minimum"), "Y Scale.Range:Maximum"=70.0 ("X Scale.Range:Minimum")) -> ()  [unwired: 2 in, 2 out]
          }
        }
        n2571 = case shown="True" "OPEN 1" {
          frame False {
          }
          frame True {
            (unwired) 0  # existing file
            w3351 = "Choose a datalog file to open"  # prompt
            n2572 = local write "OPEN 1"(FALSE ("OPEN 1")) -> ()
            n2573 = String To Path(string="C:\\LAB-IQ\\Data\\") -> (path=w3336:path)
            n2574 = File Dialog(6:"*.dgf" ("pattern"), 7:w3351, 11:w3336) -> (0:w3334:errorcluster, 3:w3342:path)  [unwired: 4 in, 2 out]
            n2575 = Unbundle(w3334) -> ()  [unwired: 3 out]
            n2576 = Strip Path(path=w3342) -> (name=w3341:string)  [unwired: 1 out]
            n2577 = Path To String(path=w3342) -> (string=w3337:string)
            "string1" <- w3337
            n2578 = Match Pattern(string=w3341, regular expression=".dgf") -> (before substring=→"String Control":string)  [unwired: 1 in, 3 out]
            n2579 = Match Pattern(string=w3337, regular expression=".dgf" ("substring (\"\")")) -> (before substring=w3347:string)  [unwired: 1 in, 3 out]
            n2580 = Concatenate Strings(w3347, ".duf" ("Substring")) -> (w3343:string)
            n2581 = String To Path(string=w3343) -> (path=w3348:path)
            n2582 = call <vilib>:"Read Characters From File.vi"("file path (dialog if empty)"=w3348, "start of read offset (chars.:0)"=60 ("start of read offset (chars.: 0)")) -> ("character string"=→"String Control 2":string)  [unwired: 4 in, 3 out]
          }
        }
        n2583 = case shown="True" "OPEN 2" {
          frame False {
          }
          frame True {
            (unwired) 0  # existing file
            w3369 = "Choose a datalog file to open"  # prompt
            n2584 = local write "OPEN 2"(FALSE ("OPEN 1")) -> ()
            n2585 = String To Path(string="C:\\LAB-IQ\\Data\\") -> (path=w3354:path)
            n2586 = File Dialog(6:"*.dgf" ("pattern"), 7:w3369, 11:w3354) -> (0:w3352:errorcluster, 3:w3360:path)  [unwired: 4 in, 2 out]
            n2587 = Unbundle(w3352) -> ()  [unwired: 3 out]
            n2588 = Strip Path(path=w3360) -> (name=w3358:string)  [unwired: 1 out]
            n2589 = Path To String(path=w3360) -> (string=w3355:string)
            "string1 2" <- w3355
            n2590 = Match Pattern(string=w3358, regular expression=".dgf") -> (before substring=→"String Control 3":string)  [unwired: 1 in, 3 out]
            n2591 = Match Pattern(string=w3355, regular expression=".dgf" ("substring (\"\")")) -> (before substring=w3366:string)  [unwired: 1 in, 3 out]
